vi "PH_Sixpack.Action Configure.vi"(0 "VI in":refnum<vi>, 5 "error in":errorcluster) -> (14 "VI out":refnum<vi>, 19 "error out":errorcluster)   [LabVIEW 2014, in "PH_Sixpack.lvlib"]
doc: "This VI is made to act on 6P hardware in a certain state. It is used in ProcPrdc."
uses:
  PH_Sixpack.lvlib
  PH_Sixpack.Status.ctl
  PH_Basics/PH_Stepmotor_BaseClass/PH_Stepmotor_BaseClass.lvlib
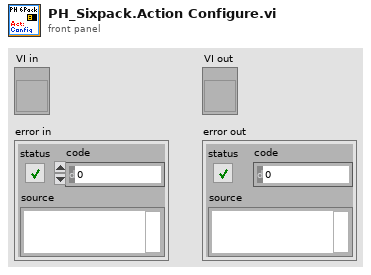
[diagram p1: front panel]
types:
  T1 = typedef "PH_Sixpack.lvlib/PH_Sixpack.Status.ctl" = enum32{"None", "Init", "Configure", "configured", "Close", "closed"}
  T2 = typedef "PH_Stepmotor_BaseClass.lvlib/PH_Stepmotor_BaseClass.i attribute.ctl" = cluster{"Device Error":errorcluster, "Axes PSDB Thread":cluster{"Ref":refnum<vi>, "Q-Ref":refnum<queue>, "Data Status":T3}, "Axes":T4[], "Axes PSDB Infos":cluster{"GUI Name":string, "PSDB Instance ID":i32, "PSDB Status Service ID":i32, "Axis":i32, "Class":string}[], "GUI Refs":T9}
  T3 = typedef "PH_PSDBWriter.lvlib/PH_PSDBWriter.Data Status.ctl" = i16
  T4 = typedef "PH_Stepmotor_BaseClass.lvlib/PH_Stepmotor_BaseClass.Axis Attributes.ctl" = cluster{"Settings":T5, "Endswitch?":bool, "DIM Service IDs":T7, "Activity":T8, "Configured?":bool, "Position":cluster{"Current":i32, "Target":i32}, "Position to set":cluster{"New?":bool, "Wanted":i32}, "Stop?":bool, "Reset?":bool, "Move?":bool, "Nothing connected?":bool}
  T5 = typedef "PH_Stepmotor_BaseClass.lvlib/PH_Stepmotor_BaseClass.Axis Settings.ctl" = cluster{"Sign change":bool, "Width":dbl, "Calibration":dbl, "Unit":string, "Motor Type":T6, "Unit Width":string, "Unit CF":string}
  T6 = typedef "PH_Stepmotor_BaseClass.lvlib/PH_Stepmotor_BaseClass.Motor Type.ctl" = enum16{"Unspecific", "OWIS 49.120.2633", "OWIS 49.060.1033", "OWIS 43.040.2558", "Diamond Motion 2200 series", "OWIS 49.120.266B.MV6", "Calorimeter", "Linear Stage 1", "MICOS VT-80", "MICOS VT-80 S", "Standa Rotstage nt0.95A", "PUF RA 320.200", "PUF RA 800.200", "PUF RA 800.400", "PUF RA 400.50", "1324.nn.800.50", "1324.n9c.800.50", "1324.nn.320.200", "1324.nn.400.200", "1324.nn.800.200", "1324.nn.400.50", "1324.8c9c.800.50", "1324.8c9c.400.200"}
  T7 = typedef "PH_Stepmotor_BaseClass.lvlib/PH_Stepmotor_BaseClass.Axis DIM Service IDs.ctl" = cluster{"Settings":i32, "Information":i32}
  T8 = typedef "PH_Stepmotor_BaseClass.lvlib/PH_Stepmotor_BaseClass.Axis Activity.ctl" = enum16{"No Information", "stopped", "running", "Failure", "Alarm", "stopped at backward ES", "stopped at foreward ES"}
  T9 = typedef "PH_Stepmotor_BaseClass.lvlib/PH_Stepmotor_BaseClass.GUI Refs.ctl" = cluster{"Axes Configuration":refnum<vi>, "Device Error":refnum<vi>, "Axes PSDB Infos":refnum<vi>}
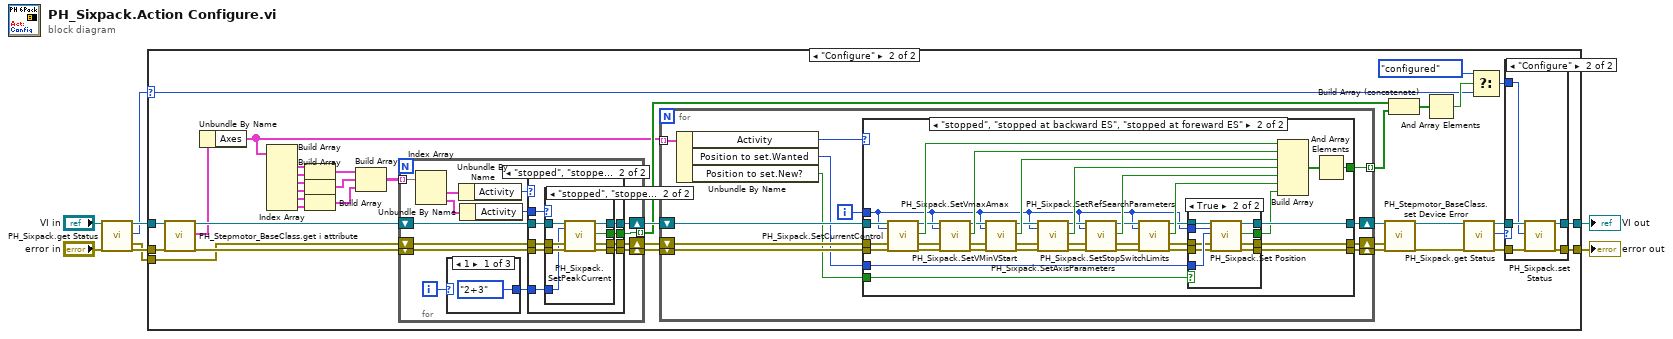
[diagram p0: block diagram]
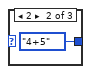
[diagram p4: hidden frame]
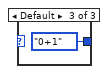
[diagram p5: hidden frame]
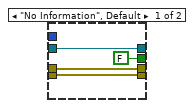
[diagram p6: hidden frame]
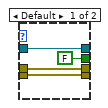
[diagram p7: hidden frame]
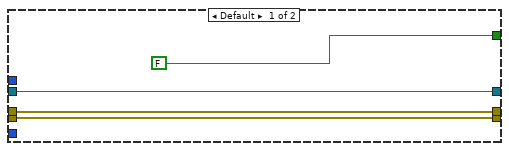
[diagram p8: hidden frame]
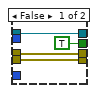
[diagram p9: hidden frame]
diagram:
  n1 = call "PH_Sixpack.get Status.vi"("VI in"="VI in", "error in (no error)"="error in") -> ("VI out"=w3:refnum<vi>, "Status"=w2:T1, "Device Error"=w1:errorcluster, "error out"=w5:errorcluster)  [unwired: 14 in]
  n2 = case shown="\"Configure\"" w2 {
    selector: w2 -> [_ w34]
    tunnel: w3 -> [w10 w44]
    tunnel: w5 -> [w9 w42]
    tunnel: [w9 w22] -> w8
    tunnel: [w10 w21] -> w7
    tunnel: w1 -> [_ w11]
    frame Default {
    }
    frame "Configure" {
      n3 = call "PH_Stepmotor_BaseClass.get i attribute.vi"("i ref in"=w44, "error in (no error)"=w42) -> ("i ref out"=w43:refnum<vi>, "i attribute"=w40:T2, "error out"=w41:errorcluster)  [unwired: 15 in]
      n4 = Unbundle By Name(w40) -> ("Axes"=w33:T4[])
      n5 = Index Array(array=w33) -> (element #1=w32:T4, element #2=w31:T4, element #3=w30:T4, element #4=w29:T4, element #5=w28:T4, element #6=w27:T4)  [unwired: 6 in]
      n6 = Build Array(w32, w31) -> (w26:T4[])
      n7 = Build Array(w30, w29) -> (w25:T4[])
      n8 = Build Array(w28, w27) -> (w24:T4[])
      n9 = Build Array(w26, w25, w24) -> (w23:T4[][])
      n10 = for {
        shift-right: [w67] -> w47
        shift-left: w41 -> [w68]
        shift-right: [w55] -> w46
        shift-left: w43 -> [w66]
        shift-right: [w64] -> w45
        shift-left: w11 -> [w65]
        tunnel: [w63] -> w38 mode=indexing
        tunnel: w23 -> [w62] mode=indexing
        i -> [w56]
        n11 = Index Array(array=w62) -> (element #1=w61:T4, element #2=w60:T4)  [unwired: 2 in]
        n12 = case shown="1" w56 {
          tunnel: [enum8{"0+1", "2+3", "4+5"}."2+3" ("MotNr (0+1)") enum8{"0+1", "2+3", "4+5"}."4+5" ("MotNr (0+1)") enum8{"0+1", "2+3", "4+5"}."0+1" ("MotNr (0+1)")] -> w57
          frame 1 {
          }
          frame 2 {
          }
          frame Default {
          }
        }
        n13 = Unbundle By Name(w61) -> ("Activity"=w58:T8)
        n14 = Unbundle By Name(w60) -> ("Activity"=w59:T8)
        n15 = case shown="\"stopped\", \"stopped at backward ES\", \"stopped at foreward ES\"" w58 {
          tunnel: w68 -> [w73 w84]
          tunnel: [w73 w83] -> w67
          tunnel: w66 -> [w75 w82]
          tunnel: [w75 w81] -> w55
          tunnel: w65 -> [w74 w80]
          tunnel: [w74 w79] -> w64
          tunnel: w57 -> [_ w78]
          tunnel: [FALSE ("ok?") w77] -> w63
          tunnel: w59 -> [_ w76]
          frame "No Information", Default {
          }
          frame "stopped", "stopped at backward ES", "stopped at foreward ES" {
            n16 = case shown="\"stopped\", \"stopped at backward ES\", \"stopped at foreward ES\"" w76 {
              tunnel: w84 -> [w86 w96]
              tunnel: [w86 w95] -> w83
              tunnel: w82 -> [w88 w94]
              tunnel: [w88 w93] -> w81
              tunnel: w80 -> [w87 w92]
              tunnel: [w87 w91] -> w79
              tunnel: w78 -> [_ w90]
              tunnel: [FALSE ("ok?") w89] -> w77
              frame Default {
              }
              frame "stopped", "stopped at backward ES", "stopped at foreward ES" {
                n17 = call "PH_Sixpack.SetPeakCurrent.vi"("i ref in"=w94, "MotNr (0+1)"=w90, "Device Error in"=w92, "error in"=w96) -> ("i ref out"=w93:refnum<vi>, "ok?"=w89:bool, "Device Error out"=w91:errorcluster, "error out"=w95:errorcluster)  [unwired: 12 in]
              }
            }
          }
        }
      }
      n18 = for {
        shift-right: [w107] -> w13
        shift-left: w46 -> [w108]
        shift-right: [w104] -> w16
        shift-left: w47 -> [w105]
        shift-right: [w102] -> w14
        shift-left: w45 -> [w103]
        tunnel: w33 -> [w101] mode=indexing
        tunnel: [w99] -> w39 mode=indexing
        i -> [w106]
        n19 = Unbundle By Name(w101) -> ("Activity"=w100:T8, "Position to set.Wanted"=w98:i32, "Position to set.New?"=w97:bool)
        n20 = case shown="\"stopped\", \"stopped at backward ES\", \"stopped at foreward ES\"" w100 {
          tunnel: w108 -> [w112 w148]
          tunnel: [w112 w119] -> w107
          tunnel: w106 -> [_ w116]
          tunnel: w105 -> [w110 w147]
          tunnel: [w110 w118] -> w104
          tunnel: w103 -> [w111 w146]
          tunnel: [w111 w117] -> w102
          tunnel: [FALSE w143] -> w99
          tunnel: w98 -> [_ w115]
          tunnel: w97 -> [_ w114]
          frame Default {
          }
          frame "stopped", "stopped at backward ES", "stopped at foreward ES" {
            n21 = call "PH_Sixpack.SetCurrentControl.vi"("i ref in"=w148, "axis"=w116, "Device Error in"=w146, "error in (no error)"=w147) -> ("i ref out"=w142:refnum<vi>, "ok?"=w145:bool, "Device Error out"=w141:errorcluster, "error out"=w140:errorcluster)  [unwired: 12 in]
            n22 = call "PH_Sixpack.SetVmaxAmax.vi"("i ref in"=w142, "axis"=w116, "Device Error in"=w141, "error in (no error)"=w140) -> ("i ref out"=w136:refnum<vi>, "ok?"=w139:bool, "Device Error out"=w137:errorcluster, "error out"=w138:errorcluster)  [unwired: 12 in]
            n23 = call "PH_Sixpack.SetVMinVStart.vi"("i ref in"=w136, "axis"=w116, "Device Error in"=w137, "error in"=w138) -> ("i ref out"=w132:refnum<vi>, "ok?"=w135:bool, "Device Error out"=w133:errorcluster, "error out"=w134:errorcluster)  [unwired: 12 in]
            n24 = call "PH_Sixpack.SetAxisParameters.vi"("i ref in"=w132, "axis"=w116, "Device Error in"=w133, "error in"=w134) -> ("i ref out"=w130:refnum<vi>, "ok?"=w131:bool, "Device Error out"=w129:errorcluster, "error out"=w128:errorcluster)  [unwired: 12 in]
            n25 = call "PH_Sixpack.SetRefSearchParameters.vi"("i ref in"=w130, "axis"=w116, "Device Error in"=w129, "error in"=w128) -> ("i ref out"=w124:refnum<vi>, "ok?"=w127:bool, "Device error out"=w125:errorcluster, "error out"=w126:errorcluster)  [unwired: 12 in]
            n26 = call "PH_Sixpack.SetStopSwitchLimits.vi"("i ref in"=w124, "axis"=w116, "Device Error in"=w125, "error in"=w126) -> ("i ref out"=w122:refnum<vi>, "ok?"=w123:bool, "Device Error out"=w120:errorcluster, "error out"=w121:errorcluster)  [unwired: 12 in]
            n27 = case shown="True" w114 {
              tunnel: w115 -> [_ w161]
              tunnel: w122 -> [w152 w160]
              tunnel: w120 -> [w151 w159]
              tunnel: w121 -> [w150 w158]
              tunnel: [w152 w157] -> w119
              tunnel: [w150 w156] -> w118
              tunnel: [w151 w155] -> w117
              tunnel: w116 -> [_ w154]
              tunnel: [TRUE ("ok?") w153] -> w113
              frame False {
              }
              frame True {
                n28 = call "PH_Sixpack.Set Position.vi"("i ref in"=w160, "axis"=w154, "Position to set"=w161, "Device Error in"=w159, "error in"=w158) -> ("i ref out"=w157:refnum<vi>, "ok?"=w153:bool, "Device Error out"=w155:errorcluster, "error out"=w156:errorcluster)  [unwired: 11 in]
              }
            }
            n29 = Build Array(w145, w139, w135, w131, w127, w123, w113) -> (w144:bool[])
            n30 = And Array Elements(Boolean array=w144) -> (logical AND=w143:bool)
          }
        }
      }
      n31 = call "PH_Stepmotor_BaseClass.set Device Error.vi"("i ref in"=w13, "Device Error"=w14, "error in"=w16) -> ("i ref out"=w12:refnum<vi>, "error out"=w15:errorcluster)  [unwired: 15 in]
      n32 = Build Array (concatenate)(w38, w39) -> (w37:bool[])
      n33 = And Array Elements(Boolean array=w37) -> (logical AND=w36:bool)
      n34 = call "PH_Sixpack.get Status.vi"("VI in"=w12, "error in (no error)"=w15) -> ("VI out"=w20:refnum<vi>, "Status"=w18:T1, "error out"=w19:errorcluster)  [unwired: 14 in, 1 out]
      n35 = Select(t=PH_Sixpack.Status."configured" ("Status in"), s=w36, f=w34) -> (s? t:f=w17:T1)
      n36 = case shown="\"Configure\"" w18 {
        tunnel: [w48 w54] -> w22
        tunnel: [w49 w53] -> w21
        tunnel: w20 -> [w49 w52]
        tunnel: w19 -> [w48 w51]
        tunnel: w17 -> [_ w50]
        frame "None", Default {
        }
        frame "Configure" {
          n37 = call "PH_Sixpack.set Status.vi"("VI in"=w52, "Status"=w50, "error in (no error)"=w51) -> ("VI out"=w53:refnum<vi>, "error out"=w54:errorcluster)  [unwired: 15 in]
        }
      }
    }
  }
  "error out" <- w8
  "VI out" <- w7
